vi "SW_Add_cage_border.vi"(10 "Bounding rectangle for outer segments, pix":T2, 11 "Picture refnum in":T1) -> (3 "Picture refnum out":T1)   [LabVIEW 2018]
uses:
  <vilib>/vision/Image Controls.llb/IMAQ Image.ctl
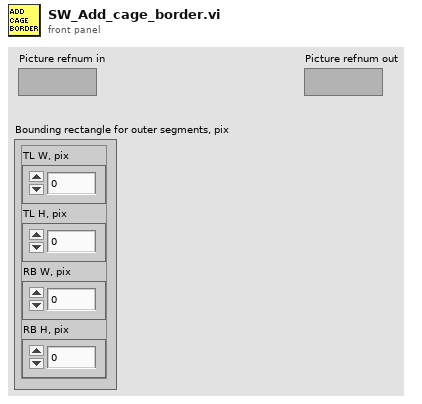
[diagram p1: front panel]
types:
  T1 = typedef "IMAQ Image.ctl" = refnum<image>
  T2 = cluster{"TL W, pix":i32, "TL H, pix":i32, "RB W, pix":i32, "RB H, pix":i32}
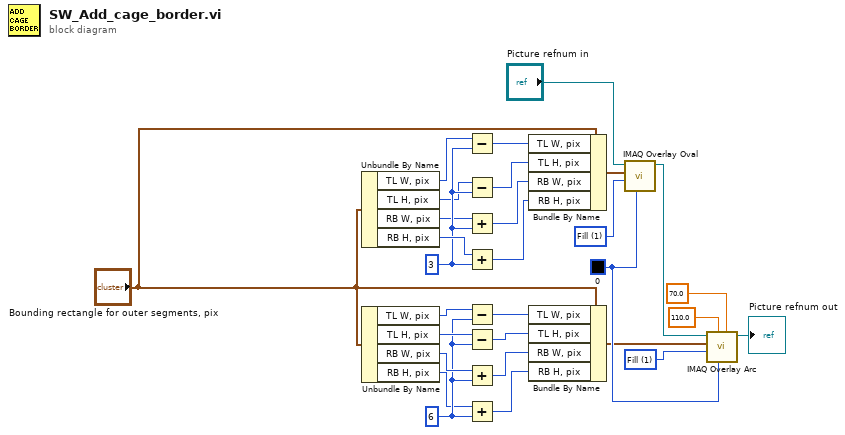
[diagram p0: block diagram]
diagram:
  w13 = u32 1 items=["Frame", "Fill"] ("Drawing Mode (Frame)")
  w20 = 6 ("y")
  w25 = u32 0 ("Color")
  w12 = u32 1 items=["Frame", "Fill"] ("Drawing Mode (Frame)")
  w4 = 3 ("y")
  n1 = Unbundle By Name("Bounding rectangle for outer segments, pix") -> ("TL W, pix"=w1:i32, "TL H, pix"=w2:i32, "RB W, pix"=w3:i32, "RB H, pix"=w5:i32)
  n2 = Unbundle By Name("Bounding rectangle for outer segments, pix") -> ("TL W, pix"=w23:i32, "TL H, pix"=w22:i32, "RB W, pix"=w21:i32, "RB H, pix"=w19:i32)
  n3 = Subtract(x=w1, y=w4) -> (x-y=w6:i32)
  n4 = Subtract(x=w2, y=w4) -> (x-y=w7:i32)
  n5 = Add(x=w3, y=w4) -> (x+y=w8:i32)
  n6 = Add(x=w5, y=w4) -> (x+y=w9:i32)
  n7 = Subtract(x=w23, y=w20) -> (x-y=w18:i32)
  n8 = Subtract(x=w22, y=w20) -> (x-y=w17:i32)
  n9 = Add(x=w21, y=w20) -> (x+y=w16:i32)
  n10 = Add(x=w19, y=w20) -> (x+y=w15:i32)
  n11 = Bundle By Name(cluster="Bounding rectangle for outer segments, pix", "TL W, pix"=w6, "TL H, pix"=w7, "RB W, pix"=w8, "RB H, pix"=w9) -> (w10:T2)
  n12 = Bundle By Name(cluster="Bounding rectangle for outer segments, pix", "TL W, pix"=w18, "TL H, pix"=w17, "RB W, pix"=w16, "RB H, pix"=w15) -> (w14:T2)
  n13 = call "IMAQ Overlay Oval"("Color"=w25, "Drawing Mode (Frame)"=w12, "Bounding Rectangle"=w10, "Image"="Picture refnum in") -> ("Image Out"=w24:T1)  [unwired: 6 in, 1 out]
  n14 = call "IMAQ Overlay Arc"("End Angle (degrees)"=70.0, "Color"=w25, "Start Angle (degrees)"=110.0, "Drawing Mode (Frame)"=w13, "Bounding Rectangle"=w14, "Image"=w24) -> ("Image Out"=→"Picture refnum out":T1)  [unwired: 4 in, 1 out]
